vi "Enable All Controls.vi"(8 "error in":errorcluster, 10 "Enable Controls":bool) -> (0 "error out":errorcluster)   [LabVIEW 2024, in "User Interface Control.lvlib"]
uses:
  User Interface Control.lvlib
  Tester Internal Communication/References - Get.vi
  Tester Internal Communication/Tester InterComm.lvlib
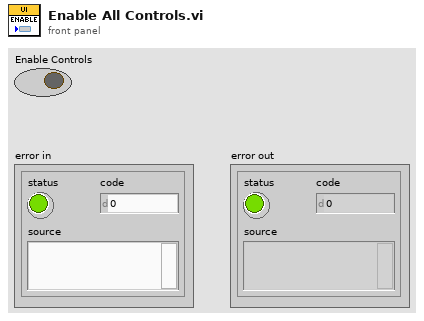
[diagram p1: front panel]
types:
  T1 = enum8{"Enabled", "Disabled", "Disabled and Grayed Out"}
  T2 = typedef "Tester InterComm.lvlib/Tester References.ctl" = cluster{"This VI":cluster{"This VI":refnum<vi>}, "UI Menu":cluster{"Tab Control":refnum<vi>, "STOP":refnum<vi>, "Working Mode":refnum<vi>}, "Indicators":cluster{"Messages Display":refnum<vi>, "Voltage Value":refnum<vi>, "PWM Value":refnum<vi>, "PWM Graph":refnum<vi>, "Duty Cycle":refnum<vi>, "Frequency":refnum<vi>, "Sinewave Graph":refnum<vi>, "ECU Connected":refnum<vi>}, "Controls":cluster{"Read Speed":refnum<vi>, "Voltage Out":refnum<vi>, "V Enable/Disable":refnum<vi>, "PWM Enable/Disable":refnum<vi>, "PWM Out":refnum<vi>, "Sine Enable/Disable":refnum<vi>, "Sinewave Out":refnum<vi>, "DO1":refnum<vi>, "DO2":refnum<vi>}}
  T3 = cluster{"Read Speed":refnum<vi>, "Voltage Out":refnum<vi>, "V Enable/Disable":refnum<vi>, "PWM Enable/Disable":refnum<vi>, "PWM Out":refnum<vi>, "Sine Enable/Disable":refnum<vi>, "Sinewave Out":refnum<vi>, "DO1":refnum<vi>, "DO2":refnum<vi>}
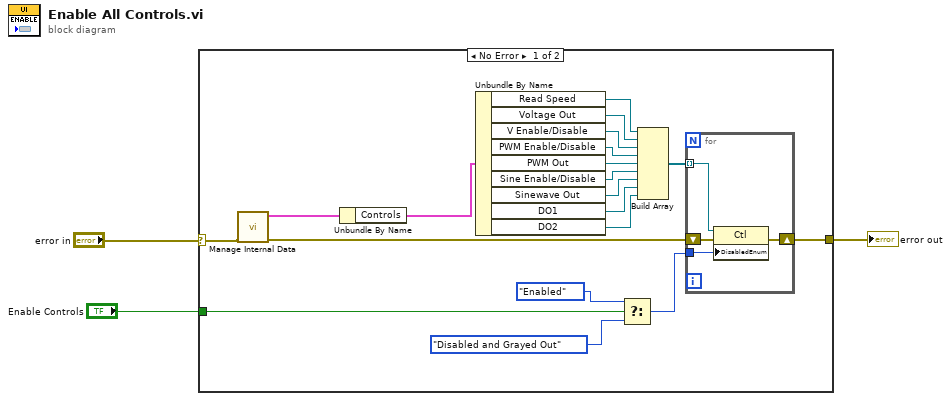
[diagram p0: block diagram]
diagram:
  n1 = case shown="No Error" "error in" {
    selector: "error in" -> [w4 w27]
    tunnel: "Enable Controls" -> [w6 _]
    tunnel: [w5 w27] -> w2
    frame No Error {
      n2 = call-poly "Manage Internal Data.vi"("error in"=w4) -> ("error out"=w10:errorcluster, "References Out"=w22:T2)  [unwired: 9 in]
      n3 = Unbundle By Name(w22) -> ("Controls"=w21:T3)
      n4 = Unbundle By Name(w21) -> ("Read Speed"=w20:refnum<vi>, "Voltage Out"=w19:refnum<vi>, "V Enable/Disable"=w18:refnum<vi>, "PWM Enable/Disable"=w17:refnum<vi>, "PWM Out"=w16:refnum<vi>, "Sine Enable/Disable"=w15:refnum<vi>, "Sinewave Out"=w14:refnum<vi>, "DO1"=w13:refnum<vi>, "DO2"=w12:refnum<vi>)
      n5 = Select(t=T1."Enabled" ("DisabledEnum"), s=w6, f=T1."Disabled and Grayed Out" ("DisabledEnum")) -> (s? t:f=w7:T1)
      n6 = Build Array(w20, w19, w18, w17, w16, w15, w14, w13, w12) -> (w11:refnum<vi>[])
      n7 = for {
        tunnel: w11 -> [w26] mode=indexing
        shift-right: [w24] -> w5
        shift-left: w10 -> [w25]
        tunnel: w7 -> [w23]
        n8 = property class="Ctl"(reference=w26, error in=w25, "DisabledEnum"=w23) -> (error out=w24:errorcluster)  [unwired: 1 out]
      }
    }
    frame Error {
    }
  }
  "error out" <- w2
